vi "Set ListSelection.vi"(8 "error in (no error)":errorcluster, 10 "BooelanValue(False)":bool, 11 "ListSelection in":refnum<class "ListSelection.lvclass">) -> (0 "error out":errorcluster, 3 "ListSelection out":refnum<class "ListSelection.lvclass">)   [LabVIEW 2015, in "Admin_Actor.lvlib" / "ListSelection.lvclass"]
uses:
  ListSelection.lvclass
  ListSelection.lvclass/ListSelection.ctl
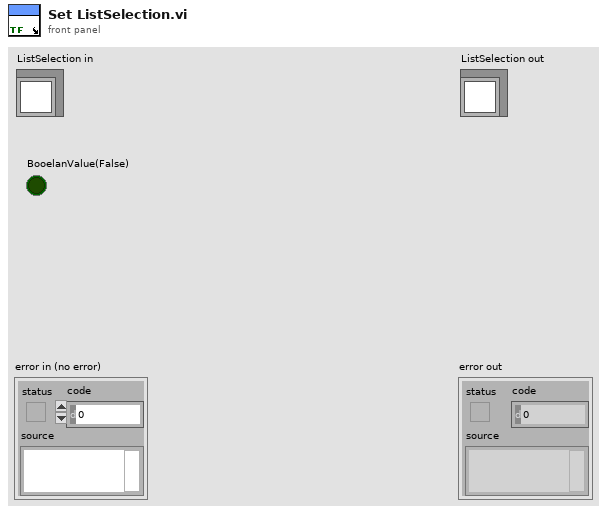
[diagram p1: front panel]
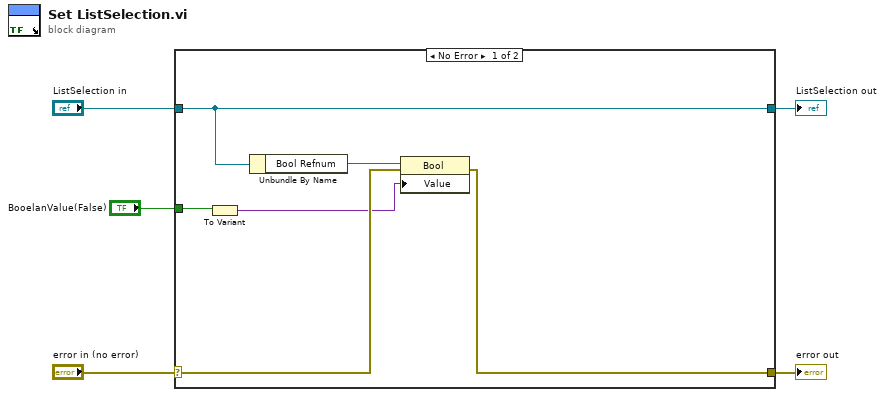
[diagram p0: block diagram]
diagram:
  n1 = case shown="No Error" "error in (no error)" {
    selector: "error in (no error)" -> [w9 w13]
    tunnel: [w8 w13] -> w4
    tunnel: [w11 w12] -> w2
    tunnel: "ListSelection in" -> [w11 w12]
    tunnel: "BooelanValue(False)" -> [w7 _]
    frame No Error {
      n2 = To Variant(anything=w7) -> (Variant=w6:variant)
      n3 = Unbundle By Name(w11) -> ("Bool Refnum"=w10:refnum<vi>)
      n4 = property class="Bool"(reference=w10, error in=w9, "Value"=w6) -> (error out=w8:errorcluster)  [unwired: 1 out]
    }
    frame Error {
    }
  }
  "error out" <- w4
  "ListSelection out" <- w2
